vi "Fdx Create Session (Generic-Board).vi"(8 "error in (no error)":errorcluster, 11 "board":u32) -> (0 "error out":errorcluster, 3 "InstrumentHandle_board out":u32, 4 "Duplicated":bool)   [LabVIEW 2020, in "AIM664LV.lvlib"]
uses:
  AIM664LV.lvlib
  _controls/hwEntry_actions.ctl
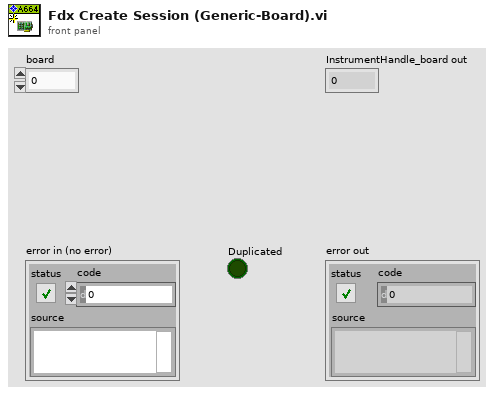
[diagram p1: front panel]
types:
  T1 = typedef "AIM664LV.lvlib/hwEntry_actions.ctl" = enum16{"Init Port", "Init Board", "Relase Port", "Release Board"}
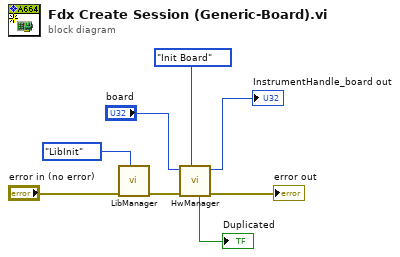
[diagram p0: block diagram]
diagram:
  n1 = call "LibManager.vi"("action"=enum16{"LibInit", "LibExit"}."LibInit", "error in (no error)"="error in (no error)") -> ("error out"=w6:errorcluster)  [unwired: 7 in, 2 out]
  n2 = call "HwManager.vi"("action (Init)"=hwEntry_actions."Init Board" ("action"), "error in (no error)"=w6, "board"="board") -> ("error out"=→"error out":errorcluster, "InstrumentHandle_board out"=→"InstrumentHandle_board out":u32, "Duplicated"=→"Duplicated":bool)  [unwired: 4 in, 2 out]
